vi "GetShooterSetpoint.vi"(10 "LimelightDistance?":bool, 11 "Setpoint":dbl) -> (3 "Setpoint Out":dbl)   [LabVIEW 2019]
uses:
  <vilib>/Rock Robotics/Network Tables/NT Read Number.vi
panel:
  in  "LookupTable Ty":cluster{"Distance":dbl, "Setpoint":dbl}[](array[cluster])=[{"Distance"=20.0, "Setpoint"=0.3}, {"Distance"=-9.65, "Setpoint"=0.3572}, {"Distance"=-18.3, "Setpoint"=0.465}, {"Distance"=-30.0, "Setpoint"=0.477}, {"Distance"=-30.0, "Setpoint"=0.477}, {"Distance"=-30.0, "Setpoint"=0.477}]
  in  "LookupTable":cluster{"Distance":dbl, "Setpoint":dbl}[](array[cluster])=[{"Distance"=0.0, "Setpoint"=0.1}, {"Distance"=91.7, "Setpoint"=0.363}, {"Distance"=120.5, "Setpoint"=0.3572}, {"Distance"=120.5, "Setpoint"=0.3572}, {"Distance"=181.3, "Setpoint"=0.465}, {"Distance"=223.3, "Setpoint"=0.477}]
  # "(In Inches for Distance)"
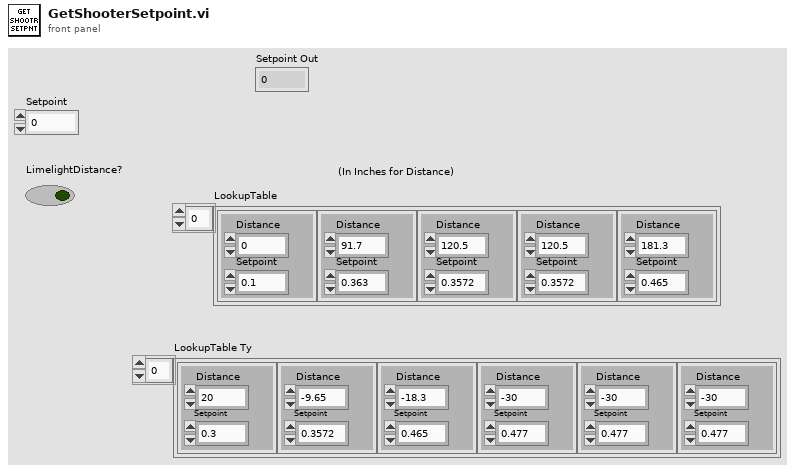
[diagram p1: front panel]
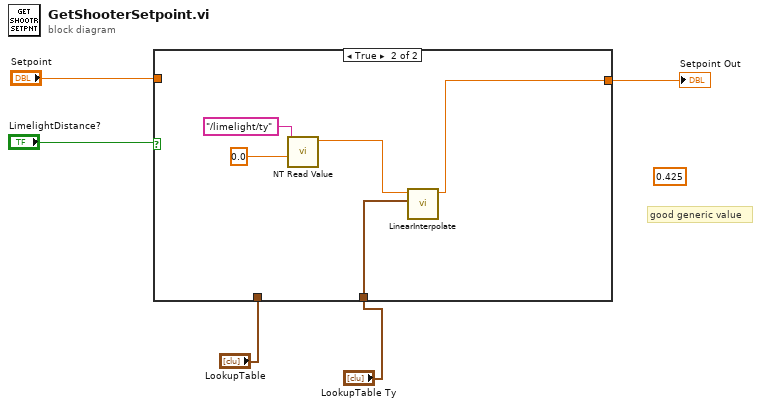
[diagram p0: block diagram]
diagram:
  (unwired) 0.425
  # "good generic value"
  n1 = case shown="True" "LimelightDistance?" {
    tunnel: [w6 w11] -> w2
    tunnel: "Setpoint" -> [w6 _]
    tunnel: "LookupTable" -> [_ _]
    tunnel: "LookupTable Ty" -> [_ w7]
    frame False {
    }
    frame True {
      n2 = call-poly <vilib>:"NT Read Value.vi"("Default Value"=0.0, "Name"="/limelight/ty") -> ("Numeric"=w8:dbl)  [unwired: 8 in, 1 out]
      n3 = call "LinearInterpolate.vi"("Points"=w7, "Value"=w8) -> ("Output"=w11:dbl)  [unwired: 9 in]
    }
  }
  "Setpoint Out" <- w2
